vi "mirrorManualMove.vi"(8 "error in (no error)":errorcluster, 10 "Ch1":sgl, 11 "Ch0":sgl) -> (0 "error out":errorcluster)   [LabVIEW 2016]
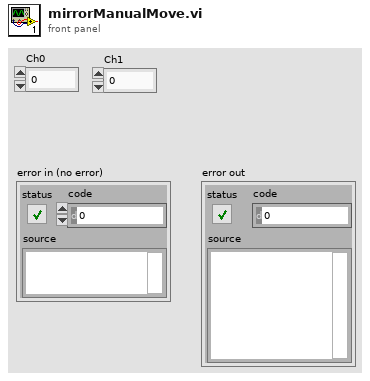
[diagram p1: front panel]
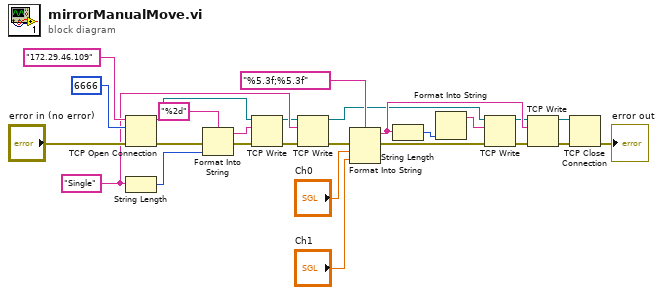
[diagram p0: block diagram]
diagram:
  w10 = "Single" ("data in")
  n1 = TCP Open Connection(address="172.29.46.109", remote port or service name=u16 6666, error in (no error)="error in (no error)") -> (connection ID=w5:refnum<k5>, error out=w9:errorcluster)  [unwired: 2 in]
  n2 = String Length(string=w10) -> (length=w11:i32)
  n3 = Format Into String(format string="%2d", error in=w9, w11) -> (resulting string=w7:string, error out=w8:errorcluster)  [unwired: 1 in]
  n4 = TCP Write(connection ID=w5, data in=w7, error in (no error)=w8) -> (connection ID out=w4:refnum<k5>, error out=w3:errorcluster)  [unwired: 1 in, 1 out]
  n5 = TCP Write(connection ID=w4, data in=w10, error in (no error)=w3) -> (connection ID out=w1:refnum<k5>, error out=w2:errorcluster)  [unwired: 1 in, 1 out]
  n6 = Format Into String(format string="%5.3f;%5.3f", error in=w2, "Ch0", "Ch1") -> (resulting string=w20:string, error out=w19:errorcluster)  [unwired: 1 in]
  n7 = String Length(string=w20) -> (length=w15:i32)
  n8 = Format Into String(w15) -> (resulting string=w14:string)  [unwired: 3 in, 1 out]
  n9 = TCP Write(connection ID=w1, data in=w14, error in (no error)=w19) -> (connection ID out=w13:refnum<k5>, error out=w12:errorcluster)  [unwired: 1 in, 1 out]
  n10 = TCP Write(connection ID=w13, data in=w20, error in (no error)=w12) -> (connection ID out=w21:refnum<k5>, error out=w22:errorcluster)  [unwired: 1 in, 1 out]
  n11 = TCP Close Connection(connection ID=w21, error in (no error)=w22) -> (error out=→"error out":errorcluster)  [unwired: 1 in, 1 out]
